vi "Get Configuration Default.vi"(8 "error in (no error)":errorcluster) -> (0 "error out":errorcluster, 3 "Measurement Configuration Default":T1)   [LabVIEW 2020, in "MeasurementTemplate_server.lvlib"]
uses:
  MeasurementTemplate_server.lvlib
  Measurement Configuration.ctl
  <vilib>/Utility/Data Type/NI_Data Type.lvlib
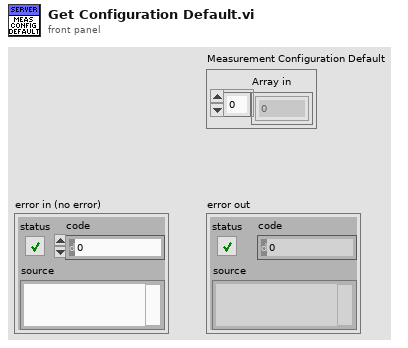
[diagram p1: front panel]
types:
  T1 = typedef "MeasurementTemplate_server.lvlib/Measurement Configuration.ctl" = cluster{"Array in":dbl[]}
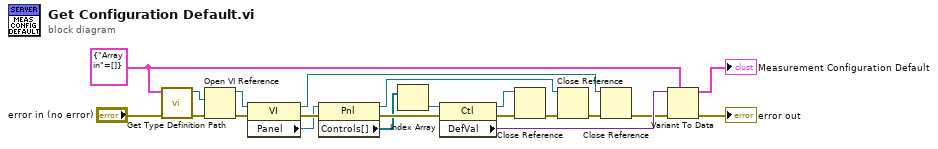
[diagram p0: block diagram]
diagram:
  w1 = T1 {"Array in"=[]} ("Measurement Configuration")
  n1 = call <vilib>:"Get Type Definition Path.vi"("error in (no error)"="error in (no error)", "variant"=w1) -> ("error out"=w17:errorcluster, "type definition path"=w6:path)  [unwired: 8 in]
  n2 = Open VI Reference(vi path=w6, error in (no error)=w17) -> (vi reference=w7:refnum<vi>, error out=w16:errorcluster)  [unwired: 4 in]
  n3 = property class="VI"(reference=w7, error in=w16) -> (reference out=w12:refnum<vi>, error out=w15:errorcluster, "Panel"=w8:refnum<vi>)
  n4 = property class="Pnl"(reference=w8, error in=w15) -> (reference out=w11:refnum<vi>, error out=w19:errorcluster, "Controls[]"=w9:refnum<vi>[])
  n5 = Index Array(array=w9) -> (element=w20:refnum<vi>)  [unwired: 1 in]
  n6 = property class="Ctl"(reference=w20, error in=w19) -> (reference out=w10:refnum<vi>, error out=w21:errorcluster, "DefVal"=w5:variant)
  n7 = Close Reference(reference=w10, error in (no error)=w21) -> (error out=w14:errorcluster)
  n8 = Close Reference(reference=w11, error in (no error)=w14) -> (error out=w13:errorcluster)
  n9 = Close Reference(reference=w12, error in (no error)=w13) -> (error out=w4:errorcluster)
  n10 = Variant To Data(error in=w4, type=w1, Variant=w5) -> (data=→"Measurement Configuration Default":T1, error out=→"error out":errorcluster)
